vi "Close Paragraph.vi"(8 "error in (no error)":errorcluster, 11 "xwpfParagraph in":refnum<class "xwpfParagraph.lvclass">) -> (0 "error out":errorcluster, 3 "xwpfParagraph out":refnum<class "xwpfParagraph.lvclass">)   [LabVIEW 2017, in "Word_Specific.lvlib" / "xwpfParagraph.lvclass"]
uses:
  xwpfParagraph.lvclass
  xwpfParagraph.lvclass/xwpfParagraph.ctl
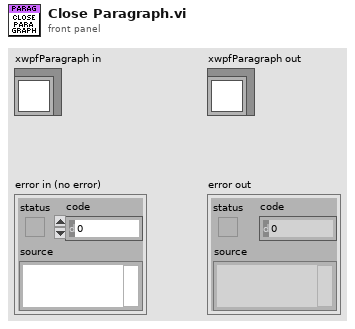
[diagram p1: front panel]
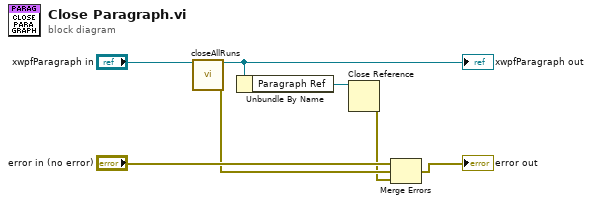
[diagram p0: block diagram]
diagram:
  n1 = call "closeAllRuns.vi"("xwpfParagraph in"="xwpfParagraph in") -> ("error out"=w2:errorcluster, "xwpfParagraph out"=w3:refnum<class "xwpfParagraph.lvclass">)  [unwired: 9 in]
  "xwpfParagraph out" <- w3
  n2 = Unbundle By Name(w3) -> ("Paragraph Ref"=w6:refnum<k24>)
  n3 = Close Reference(reference=w6) -> (error out=w1:errorcluster)  [unwired: 1 in]
  n4 = Merge Errors("error in (no error)", w2, w1) -> (→"error out":errorcluster)
